vi "consumer.vi"() -> ()   [LabVIEW 2020]
uses:
  <userlib>/Zaphiro/GTools/Redis/Sources/Redis/Redis.lvclass/Redis.ctl
  aea59807-97c7-47ab-b578-198c3bfad1a9.vi
  f854457d-36a3-4227-beff-9843280818cc.vi
  b567c38f-e722-4316-83bf-2d80707c7bfa.vi
  <userlib>/Zaphiro/GTools/Redis/Sources/Redis/Connection/PING.vi
  aea59807-97c7-47ab-b578-198c3bfad1a9.vi/7c7783df-fd5a-49d9-9b7a-63cc9fb0e4e5.vi
  <userlib>/Zaphiro/GTools/Redis/Sources/Redis/Connection/QUIT.vi
  <userlib>/Zaphiro/GTools/Redis/Sources/Redis/subVIs/LL_collect-response.vi
  <userlib>/Zaphiro/GTools/Redis/Sources/Redis/Redis.lvclass
  <vilib>/Comparison/Less/Less Functor/Less Functor.lvclass
panel:
  in  "lb-meas":i32[](listbox) caption="Available measurements"
  out "values":string[](array[string])
  out "measurements":string[](array[string])
  in  "lb-ts":i32(listbox) caption="Available HASH (timestamps)"
  in  "check-ts":bool
  in  "check-list":bool
  in  "connection":cluster{"ip":string, "port":u16, "timeout":i32}={"ip"="localhost", "port"=6379, "timeout"=1000}
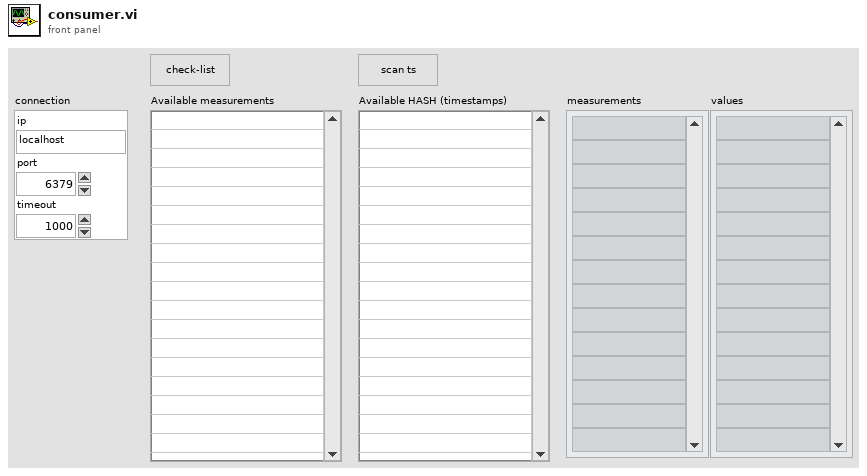
[diagram p1: front panel]
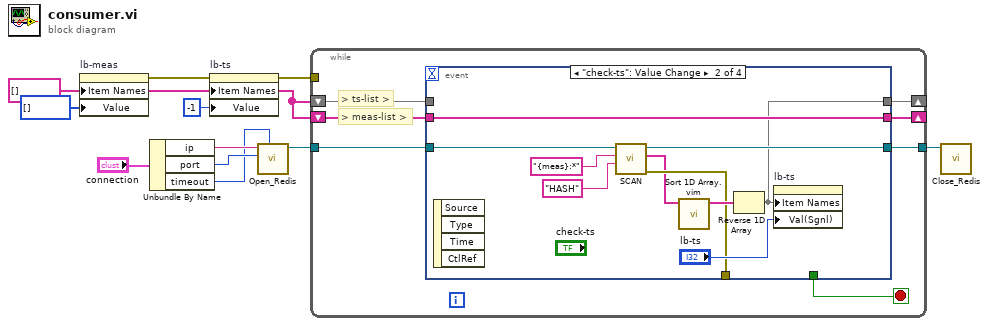
[diagram p0: block diagram]
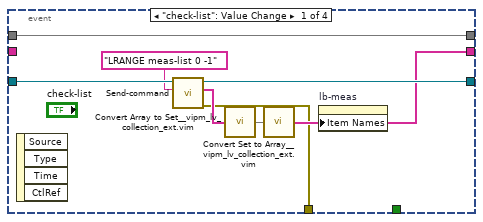
[diagram p2: hidden frame]
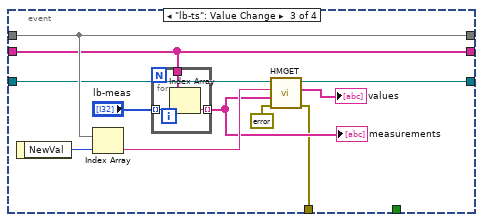
[diagram p3: hidden frame]
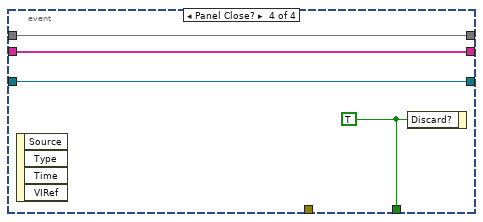
[diagram p4: hidden frame]
diagram:
  w1 = string[] [] ("Item Names")
  n1 = property on="lb-meas" class="LstBox (strict)"("Item Names"=w1, "Value"=i32[] [] ("lb-meas")) -> (error out=w2:errorcluster)  [unwired: 2 in, 1 out]
  n2 = Unbundle By Name("connection") -> ("ip"=w10:string, "port"=w9:u16, "timeout"=w8:i32)
  n3 = property on="lb-ts" class="LstBox (strict)"(error in=w2, "Item Names"=w1, "Value"=-1 ("available timestamps")) -> (error out=w5:errorcluster)  [unwired: 1 in, 1 out]
  n4 = call <userlib>:"Open_Redis.vi"("Tcp timeout ms"=w8, "Port"=w9, "Host"=w10) -> ("output cluster"=w7:refnum<class "Redis.lvclass">)  [unwired: 6 in, 2 out]
  n5 = while {
    tunnel: w7 -> [w18]
    tunnel: [w17] -> w6
    shift-right: [w15] -> _
    shift-left: w1 -> [w14]
    shift-right: [w13] -> _
    shift-left: w1 -> [w12]
    tunnel: w5 -> [_]
    stop <- w16 stop-if-true
    # "> ts-list >"
    # "> meas-list >"
    n6 = event shown="[1] \"check-ts\": Value Change" {
      selector: _ -> [_ _ _ _]
      dyn-events: _ -> [_ _ _ _]
      timeout: _ -> [_ _ _ _]
      tunnel: w18 -> [w26 w35 w45 w53]
      tunnel: [w25 w34 w46 w53] -> w17
      tunnel: [_ _ _ w54] -> w16
      tunnel: [w20 w36 w39 w52] -> w15
      tunnel: w14 -> [_ w36 w39 w52]
      tunnel: [w21 w27 w47 w51] -> w13
      tunnel: w12 -> [w21 _ w47 w51]
      tunnel: [w19 w29 w37 _] -> _
      event "check-list": Value Change {
        n7 = event-data() -> ()  [unwired: 1 in, 4 out]
        n8 = call <userlib>:"Send-command.vi"("command"="LRANGE meas-list 0 -1" ("Key"), "Redis.lvclass in"=w26) -> ("error out"=w19:errorcluster, "redis reply"=w22:string[], "Redis.lvclass out"=w25:refnum<class "Redis.lvclass">)  [unwired: 7 in]
        n9 = call "Convert Array to Set__vipm_lv_collection_ext.vim"("array"=w22) -> ("set"=w23:set{string})  [unwired: 6 in]
        n10 = call "Convert Set to Array__vipm_lv_collection_ext.vim"("set"=w23) -> ("array"=w20:string[])  [unwired: 8 in]
        n11 = property on="lb-meas" class="LstBox (strict)"("Item Names"=w20) -> ()  [unwired: 2 in, 2 out]
      }
      event "check-ts": Value Change {
        n12 = event-data() -> ()  [unwired: 1 in, 4 out]
        n13 = call <userlib>:"SCAN.vi"("Type"="HASH" ("Key"), "Pattern"="{meas}:*" ("Key"), "Redis.lvclass in"=w35) -> ("error out"=w29:errorcluster, "redis reply"=w28:string[], "Redis.lvclass out"=w34:refnum<class "Redis.lvclass">)  [unwired: 6 in]
        n14 = call "Sort 1D Array.vim"("unsorted array"=w28) -> ("sorted array"=w31:string[])  [unwired: 10 in]
        n15 = Reverse 1D Array(array=w31) -> (reversed array=w27:string[])
        n16 = property on="lb-ts" class="LstBox (strict)"("Item Names"=w27, "Val(Sgnl)"="lb-ts") -> ()  [unwired: 2 in, 2 out]
      }
      event "lb-ts": Value Change {
        n17 = event-data() -> ("NewVal"=w41:i32)  [unwired: 1 in]
        n18 = Index Array(array=w47, index=w41) -> (element=w44:string)
        n19 = for {
          tunnel: "lb-meas" -> [w49] mode=indexing
          tunnel: w39 -> [w50]
          tunnel: [w48] -> w38 mode=indexing
          n20 = Index Array(array=w50, index=w49) -> (element=w48:string)
        }
        "measurements" <- w38
        n21 = call <userlib>:"HMGET.vi"("error in"=errorcluster {"status"=FALSE, "code"=0, "source"=""}, "Fields"=w38, "Key"=w44, "Redis.lvclass in"=w45) -> ("error out"=w37:errorcluster, "redis reply"=→"values":string[], "Redis.lvclass out"=w46:refnum<class "Redis.lvclass">)  [unwired: 5 in]
      }
      event Panel Close? {
        w54 = TRUE ("Discard?")
        n22 = event-data() -> ()  [unwired: 1 in, 4 out]
        n23 = event-data("Discard?"=w54) -> ()  [unwired: 1 in, 1 out]
      }
    }
  }
  n24 = call <userlib>:"Close_Redis.vi"("Redis.lvclass in"=w6) -> ()  [unwired: 9 in, 2 out]
